vi "(PPMS) Manual Build.vi"(11 "Path to VIPB File":path=path "C:/Users/patrick/Documents/GitHub/PPMS-Monitor-and-Control/build support/PPMS Instrument.vipb") -> ()   [LabVIEW 2019]
uses:
  <userlib>/LevyLab/Build Support/ProgressBar/ProgressBar.lvclass
  <vilib>/AppBuilder/AB_API_Simple/Build Specification Version.ctl
  <vilib>/AppBuilder/AB_API_Simple/Set Build Specification Version (path).vi
  <vilib>/AppBuilder/AB_API_Simple/Build (path).vi
  <vilib>/AppBuilder/AB_API_Simple/NI_App_Builder_API.lvlib
  <vilib>/JKI/VIPM API/VIPM API_vipm_api.lvlib
  <userlib>/LevyLab/Build Support/PostBuildSupport/PostBuildSupport.lvclass
panel:
  out "Current State":string="Exit"
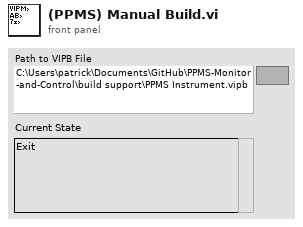
[diagram p1: front panel]
types:
  T1 = enum32{"Invalid", "Standard", "Closed", "Hidden", "Minimized", "Maximized"}
  T2 = enum32{"invalid app kind", "Development System", "Run Time System", "Student Edition", "Embedded LabVIEW", "Evaluation", "Custom"}
  T3 = typedef "NI_App_Builder_API.lvlib/Build Specification Version.ctl" = cluster{"Major":u16, "Minor":u16, "Fix":u16, "Build":u16}
  T4 = cluster{"Core":cluster{"Current VI Reference":refnum<vi>, "Close Panel on Exit?":bool}, "ProgressBar":refnum<class "ProgressBar.lvclass">, "Product Name":string, "Package Version":string, "Package Source Folder":path, "Path to Project":path, "Path to VIPB File":path, "Output Package File Path":path}
  T5 = cluster{"Current VI Reference":refnum<vi>, "Close Panel on Exit?":bool}
  T6 = typedef "VIPM API_vipm_api.lvlib/VI Package Build Spec Data Cluster_vipm_api.ctl" = cluster{"Package Version":T7, "Product Name":string, "Company Name":string, "Author Name (Person or Company)":string, "Product Homepage (URL)":string, "Legal Copyright":string, "License Agreement Name":string, "Product Description Summary":string, "Product Description":string, "Release Notes - Change Log":string}
  T7 = typedef "VIPM API_vipm_api.lvlib/Version Info Cluster_vipm_api.ctl" = cluster{"major":u32, "minor":u32, "patch":u32, "build":u32}
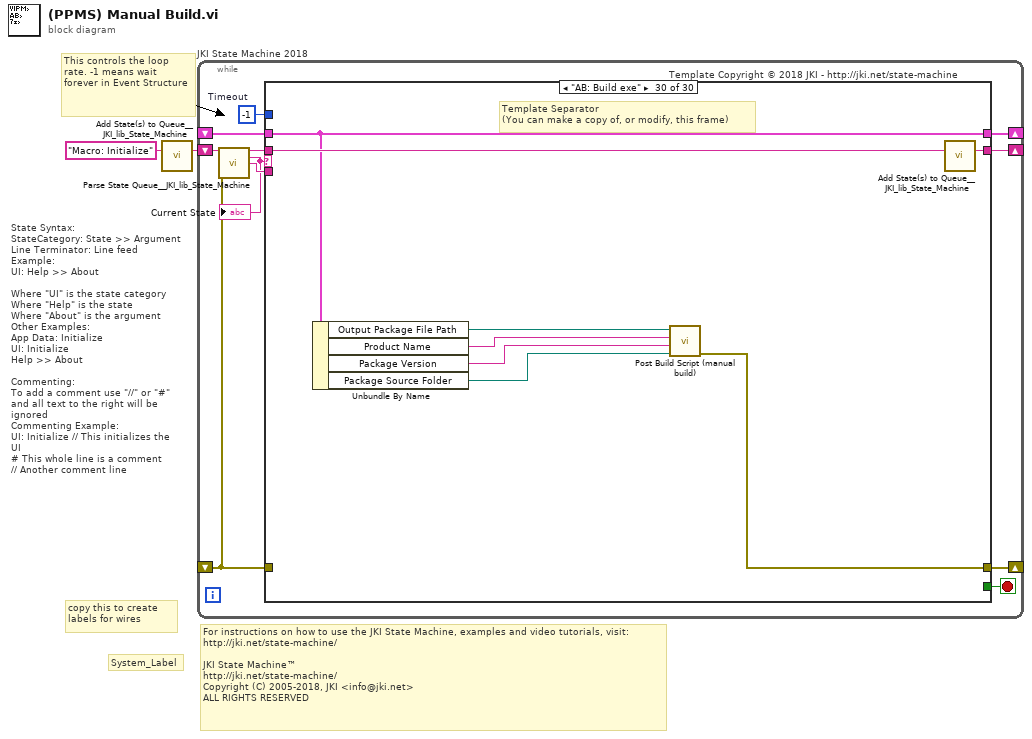
[diagram p0: block diagram]
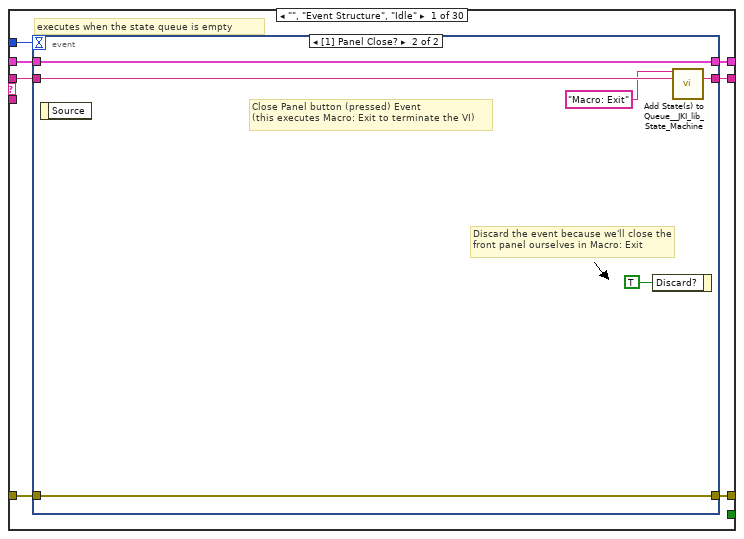
[diagram p2: hidden frame]
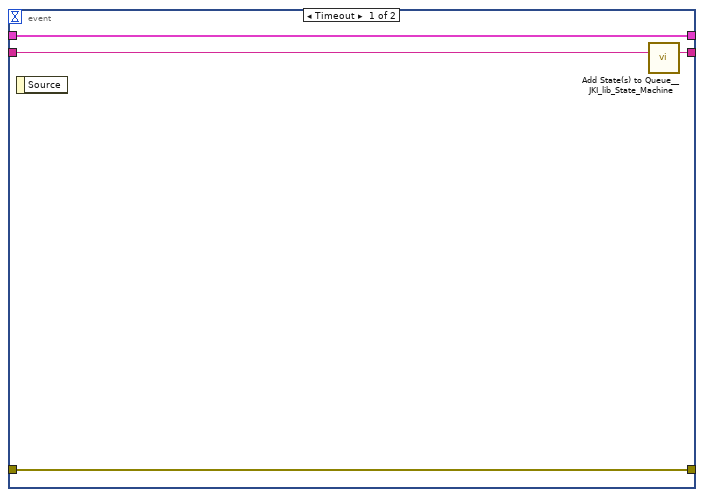
[diagram p3: hidden frame]
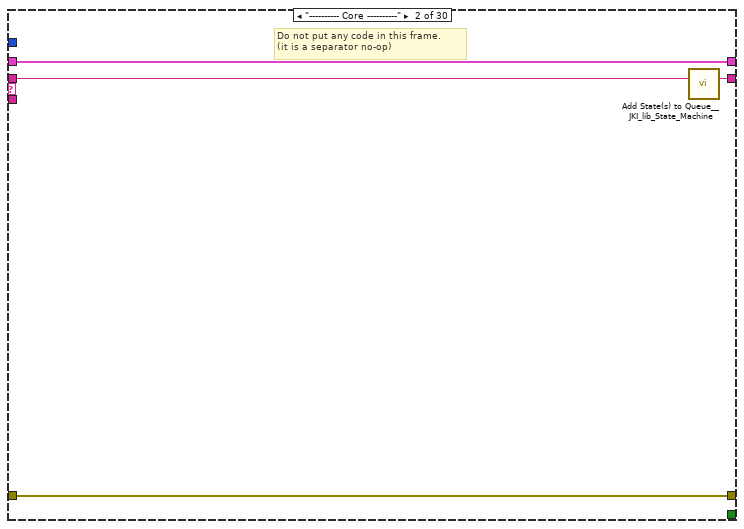
[diagram p4: hidden frame]
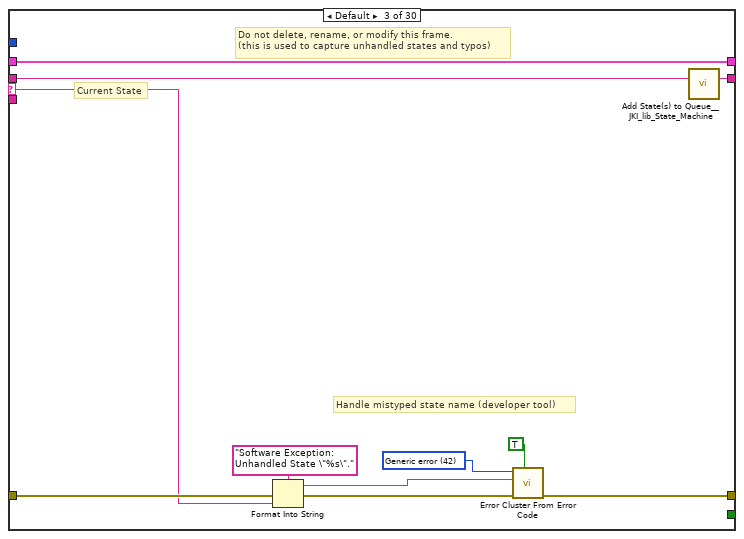
[diagram p5: hidden frame]
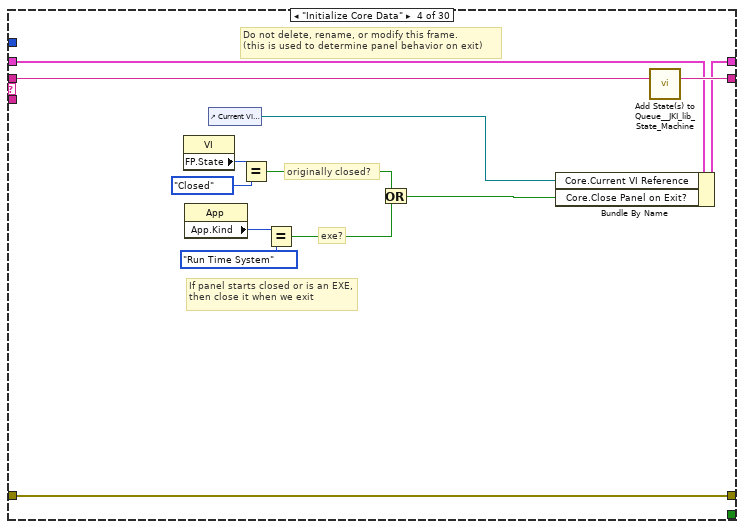
[diagram p6: hidden frame]
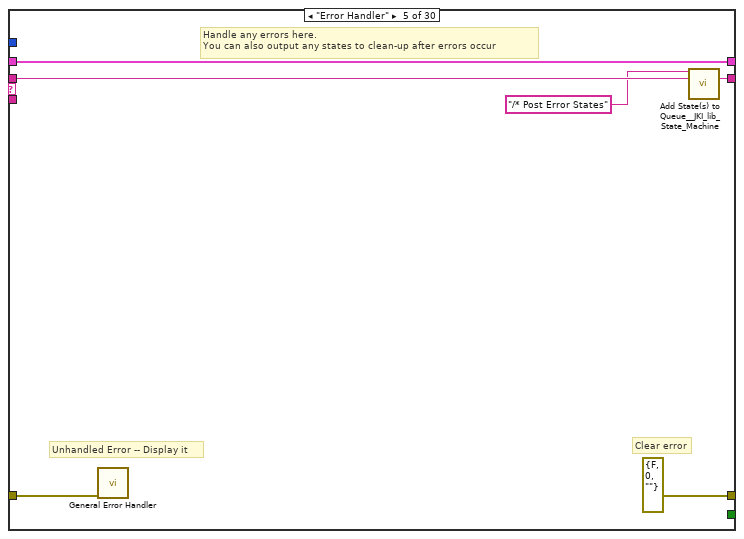
[diagram p7: hidden frame]
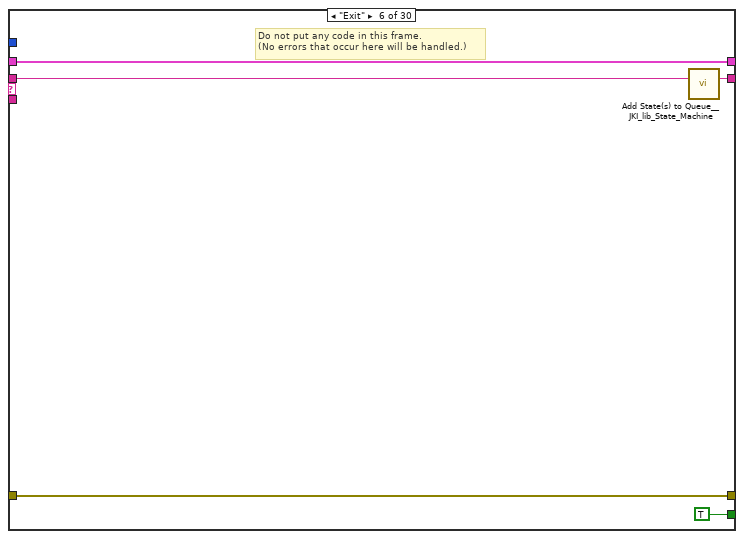
[diagram p8: hidden frame]
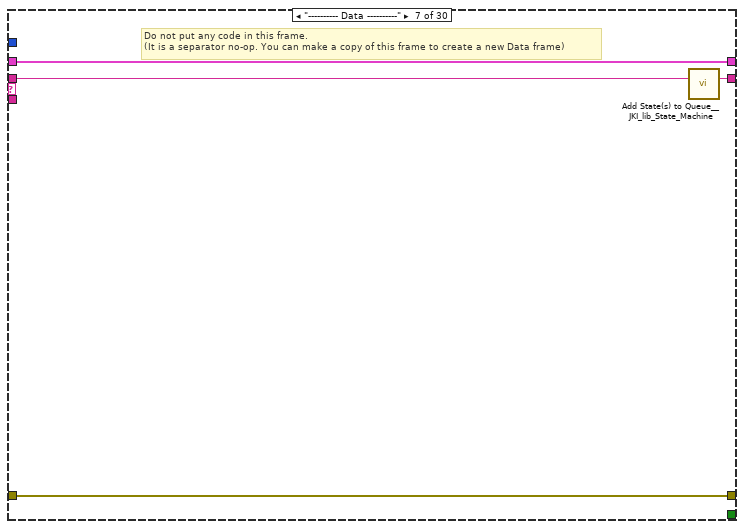
[diagram p9: hidden frame]
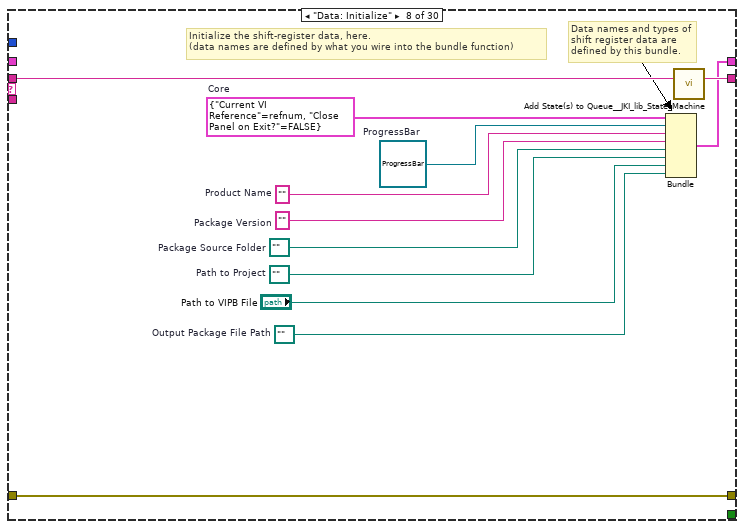
[diagram p10: hidden frame]
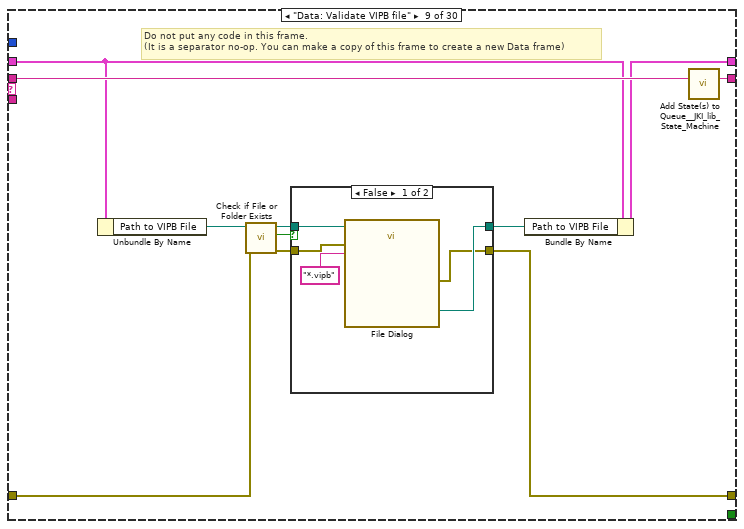
[diagram p11: hidden frame]
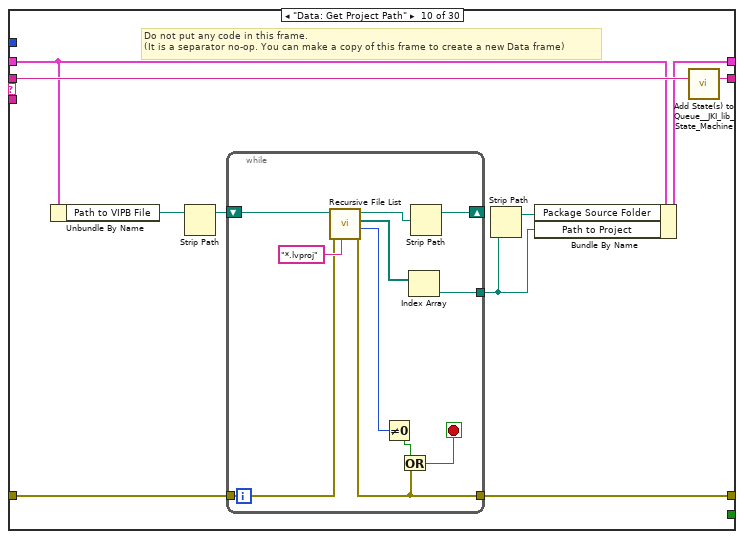
[diagram p13: hidden frame]
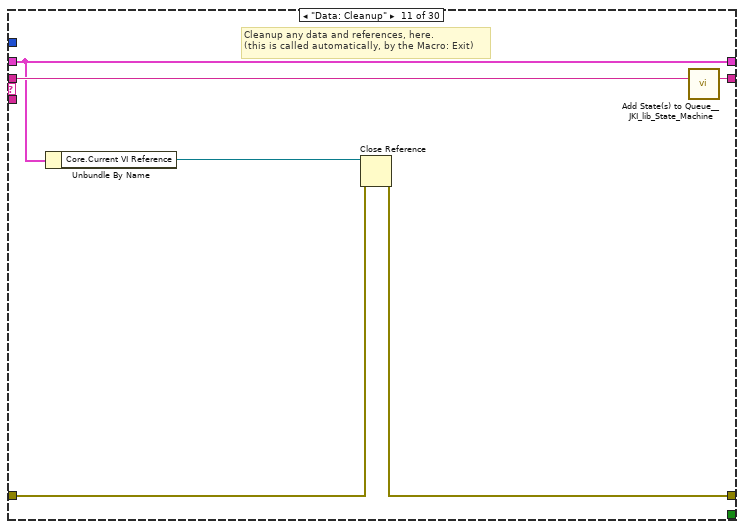
[diagram p14: hidden frame]
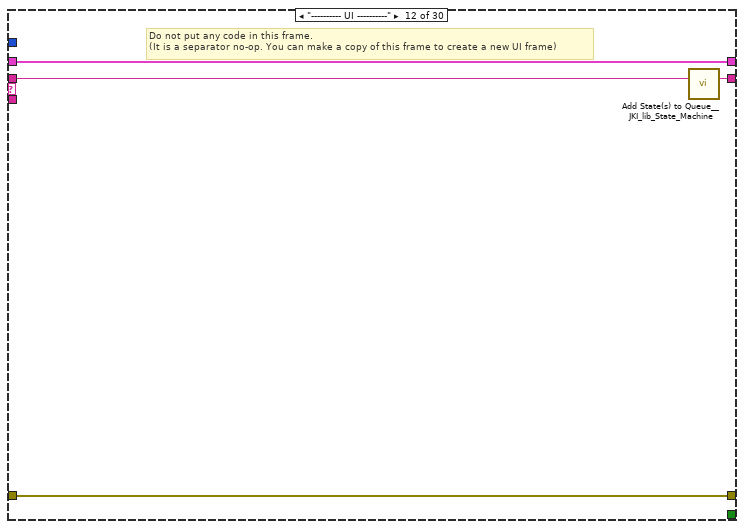
[diagram p15: hidden frame]
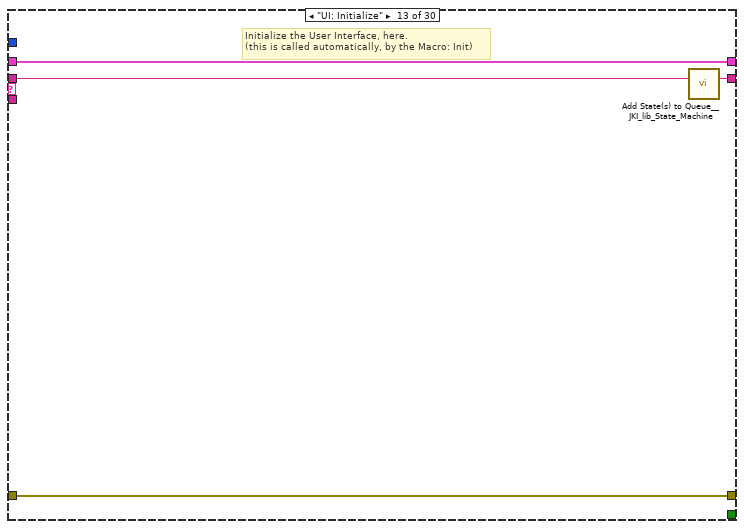
[diagram p16: hidden frame]
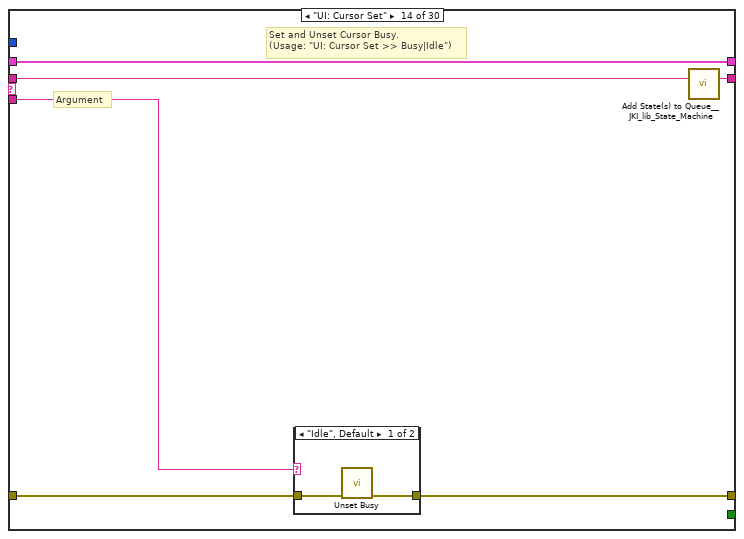
[diagram p17: hidden frame]
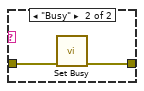
[diagram p18: hidden frame]
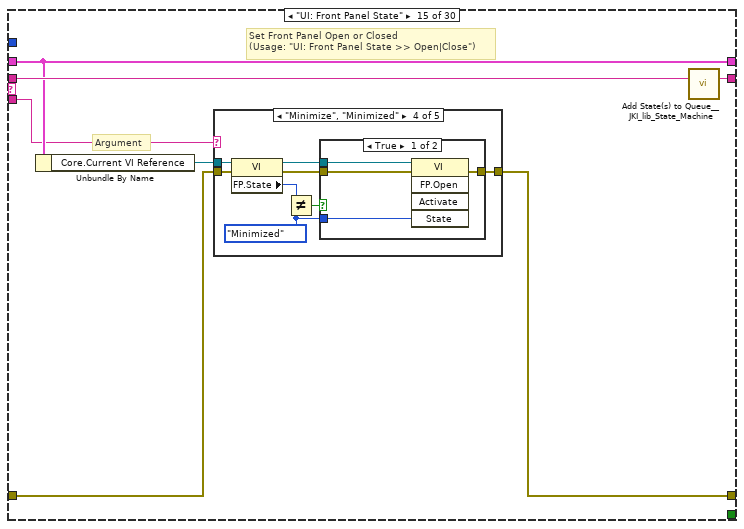
[diagram p19: hidden frame]
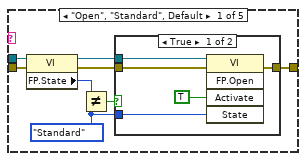
[diagram p20: hidden frame]
diagram:
  # "For instructions on how to use the JKI State Machine, examples and video tutorials, visit:\nhttp://jki.net/state-machine/\n\nJKI State Machine™\nhttp://jki.net/state-machine/\nCopyright (C) 2005-2018, JKI <info@jki.net>\nALL RIGHTS RESERVED"
  # "State Syntax:\nStateCategory: State >> Argument\nLine Terminator: Line feed\nExample:\nUI: Help >> About\n\nWhere \"UI\" is the state category\nWhere \"Help\" is the state\nWhere \"About\" is the argument\nOther Examples:\nApp Data: Initialize\nUI: Initialize\nHelp >> About\n\nCommenting:\nTo add a comment use \"//\" or \"#\" and all text to the right will be ignored\nCommenting Example:\nUI: Initialize // This initializes the UI\n# This whole line is a comment\n// Another comment line"
  # "copy this to create labels for wires"
  # "This controls the loop rate. -1 means wait forever in Event Structure"
  # "System_Label"
  n1 = call <vilib>:"Add State(s) to Queue__JKI_lib_State_Machine.vi"("State(s) in (\"\")"="Macro: Initialize") -> ("States Out"=w2:string)  [unwired: 14 in]
  n2 = while "JKI State Machine 2018" {
    shift-right: [w7] -> _
    shift-left: _ -> [w6]
    shift-right: [w10] -> _
    shift-left: _ -> [w4]
    shift-right: [w9] -> _
    shift-left: w2 -> [w11]
    stop <- w8 stop-if-true
    w5 = -1  # Timeout
    # "Template Copyright © 2018 JKI - http://jki.net/state-machine"
    n3 = call <vilib>:"Parse State Queue__JKI_lib_State_Machine.vi"("State Queue"=w11, "Error In (no error)"=w4) -> ("Remaining States"=w13:string, "Current State"=w3:string, "Arguments"=w12:string)  [unwired: 11 in]
    "Current State" <- w3
    n4 = case shown="\"AB: Build exe\"" w3 {
      selector: w3 -> [_ _ w35 _ _ _ _ _ _ _ _ _ _ _ _ _ _ _ _ _ _ _ _ _ _ _ _ _ w327 _]
      tunnel: w13 -> [w20 w34 w39 w58 w64 w69 w73 w85 w96 w113 w130 w134 w138 w144 w155 w224 w229 w234 w245 w249 w265 w273 w277 w285 w293 w302 w306 w324 w337 w345]
      tunnel: w12 -> [_ _ _ _ _ _ _ _ _ _ _ _ _ w139 w149 _ _ _ _ _ _ _ _ _ _ w294 _ w319 w328 _]
      tunnel: w6 -> [w18 w31 w37 w51 w61 w67 w70 _ w89 w110 w125 w131 w136 w142 w151 w221 w226 w231 w242 w247 w255 w266 w275 w278 w290 w299 w304 w322 w335 w343]
      tunnel: [w17 w32 w41 w55 errorcluster {"status"=FALSE, "code"=0, "source"=""} ("error out") w66 w71 w82 w88 w109 w126 w132 w135 w140 w152 w222 w227 w232 w243 w246 w252 w270 w274 w281 w286 w296 w303 w309 w332 w339] -> w10
      tunnel: w4 -> [w16 w32 w40 w55 w60 w66 w71 w82 w86 w108 w127 w132 w135 w141 w153 w222 w227 w232 w243 w246 w254 w269 w274 w280 w287 w295 w303 w307 w330 _]
      tunnel: [w19 w33 w38 w57 w63 w68 w72 w84 w95 w112 w129 w133 w137 w143 w154 w223 w228 w233 w244 w248 w264 w272 w276 w284 w292 w301 w305 w323 w336 w344] -> w9
      tunnel: [_ _ _ _ _ TRUE _ _ _ _ _ _ _ _ _ _ _ _ _ _ _ _ _ _ _ _ _ _ _ _] -> w8
      tunnel: [w15 w31 w37 w56 w61 w67 w70 w83 w90 w111 w125 w131 w136 w142 w151 w221 w226 w231 w242 w247 w256 w267 w275 w279 w291 w300 w304 w322 w335 w343] -> w7
      tunnel: w5 -> [w14 _ _ _ _ _ _ _ _ _ _ _ _ _ _ _ _ _ _ _ _ _ _ _ _ _ _ _ _ _]
      frame "", "Event Structure", "Idle" {
        # "executes when the state queue is empty"
        n5 = event shown="[1] Panel Close?" {
          selector: _ -> [_ _]
          dyn-events: _ -> [_ _]
          timeout: w14 -> [_ _]
          tunnel: w20 -> [w24 w30]
          tunnel: [w23 w29] -> w19
          tunnel: w18 -> [w21 w27]
          tunnel: [w22 w28] -> w17
          tunnel: w16 -> [w22 w28]
          tunnel: [w21 w27] -> w15
          event Timeout {
            n6 = event-data() -> ()  [unwired: 1 in, 1 out]
            n7 = call <vilib>:"Add State(s) to Queue__JKI_lib_State_Machine.vi"("State(s) in (\"\")"=w24) -> ("States Out"=w23:string)  [unwired: 14 in]
          }
          event Panel Close? {
            # "Discard the event because we'll close the front panel ourselves in Macro: Exit"
            # "Close Panel button (pressed) Event\n(this executes Macro: Exit to terminate the VI)"
            n8 = event-data() -> ()  [unwired: 1 in, 1 out]
            n9 = event-data("Discard?"=TRUE) -> ()  [unwired: 1 in, 1 out]
            n10 = call <vilib>:"Add State(s) to Queue__JKI_lib_State_Machine.vi"("State(s) in Front (\"\")"="Macro: Exit", "State(s) in (\"\")"=w30) -> ("States Out"=w29:string)  [unwired: 13 in]
          }
        }
      }
      frame "---------- Core ----------" {
        # "Do not put any code in this frame.\n(it is a separator no-op)"
        n11 = call <vilib>:"Add State(s) to Queue__JKI_lib_State_Machine.vi"("State(s) in (\"\")"=w34) -> ("States Out"=w33:string)  [unwired: 14 in]
      }
      frame Default {
        w44 = 42 items=["No error", "Argument error", "Memory is full", "Out of zone", "End of file", "File already open", "Generic file I/O error", "File not found", "File permission error", "Disk is full", "Duplicate path", "Too many files open", "System feature not enabled", "Resource file not found", "Cannot add resource", "Resource not found", "Image not found", "Image memory error", "Pen does not exist", "Config type invalid", "Config token not found", "Config parse error", "Config memory error", "Bad external code format", "Bad external code offset", "External code not present", "Null window", "Destroy window error", "Null menu", "Print aborted", "Bad print record", "Print driver error", "Windows error during printing", "Memory error during printing", "Print dialog error", "Generic print error", "Invalid device refnum", "Device not found", "Device parameter error", "Device unit error", "Cannot open device", "Device call aborted", "Generic error", "Cancelled by user", "Object ID too low", "Object ID too high", "Object not in heap", "Unknown heap", "Unknown object (invalid DefProc)", "Unknown object (DefProc not in table)", "Message out of range", "Invalid (null) method", "Unknown message", "Manager call not supported", "Bad address", "Network operation in progress", "Network operation timed out", "Connection is busy", "Network attribute not supported", "Network error", "Address in use", "System out of memory", "Connection aborted", "Connection refused", "Not connected", "Already connected", "Connection closed", "Initialization error (interapplication manager)", "Bad occurrence", "Wait on unbound occurrence handler", "Occurrence queue overflow", "Datalog type conflict", "Unused", "Unrecognized type (interapplication manager)", "Memory corrupt", "Failed to make temporary DLL", "Old CIN version", "Drag socket not found", "Failed to load drop-object", "Failed to register OLE object", "Failed to release OLE object", "Format specifier type mismatch", "Unknown format specifier", "Too few format specifiers", "Too many format specifiers", "Scan failed", "Newer CIN version", "Error converting to variant", "Runtime menu error", "Password tampered", "Variant attribute not found", "Incompatible variant data type", "Event data is not available", "Event Store is not present", "Occurrence is not found", "Event Queue is not created", "Event info is not available", "Refnum passed is NULL", "Error retrieving Class GUID", "Error retrieving CoClass GUID", "Error retrieving TypeLib GUID.", "Bad built application magic bytes.", "Specific driver is different from the specific driver associated with the Logical Name.", "There is no session opened to the class driver.", "Max Error", "MAX - Error with config objects", "MAX - Error loading configuration", "MAX - Group not supported"]
        # "Current State"
        # "Do not delete, rename, or modify this frame.\n(this is used to capture unhandled states and typos)"
        # "Handle mistyped state name (developer tool)"
        n12 = Format Into String(format string="Software Exception: Unhandled State \"%s\"." ("message"), error in=w40, w35) -> (resulting string=w43:string, error out=w42:errorcluster)  [unwired: 1 in]
        n13 = call <vilib>:"Error Cluster From Error Code.vi"("show call chain? (False)"=TRUE, "error in (no error)"=w42, "error message (\"\")"=w43, "error code (0)"=w44) -> ("error out"=w41:errorcluster)  [unwired: 5 in]
        n14 = call <vilib>:"Add State(s) to Queue__JKI_lib_State_Machine.vi"("State(s) in (\"\")"=w39) -> ("States Out"=w38:string)  [unwired: 14 in]
      }
      frame "Initialize Core Data" {
        # "Do not delete, rename, or modify this frame.\n(this is used to determine panel behavior on exit)"
        # "originally closed?"
        # "exe?"
        # "If panel starts closed or is an EXE, then close it when we exit"
        n15 = property class="VI"() -> ("FP.State"=w48:T1)  [unwired: 2 in, 2 out]
        n16 = property class="App"() -> ("App.Kind"=w54:T2)  [unwired: 2 in, 2 out]
        n17 = control-ref of="Current VI Reference"() -> (w49:refnum<vi>)
        n18 = Equal?(x=w48, y=T1."Closed" ("Front Panel Window:State")) -> (x = y?=w46:bool)
        n19 = Equal?(x=w54, y=T2."Run Time System" ("Application:Kind")) -> (x = y?=w52:bool)
        n20 = Or(x=w46, y=w52) -> (x .or. y?=w50:bool)
        n21 = Bundle By Name(cluster=w51, "Core.Current VI Reference"=w49, "Core.Close Panel on Exit?"=w50) -> (w56:T4)
        n22 = call <vilib>:"Add State(s) to Queue__JKI_lib_State_Machine.vi"("State(s) in (\"\")"=w58) -> ("States Out"=w57:string)  [unwired: 14 in]
      }
      frame "Error Handler" {
        # "Unhandled Error -- Display it"
        # "Handle any errors here.\nYou can also output any states to clean-up after errors occur"
        # "Clear error"
        n23 = call <vilib>:"General Error Handler.vi"("error in (no error)"=w60) -> ()  [unwired: 10 in, 5 out]
        n24 = call <vilib>:"Add State(s) to Queue__JKI_lib_State_Machine.vi"("State(s) in Front (\"\")"="/* Post Error States", "State(s) in (\"\")"=w64) -> ("States Out"=w63:string)  [unwired: 13 in]
      }
      frame "Exit" {
        # "Do not put any code in this frame.\n(No errors that occur here will be handled.)"
        n25 = call <vilib>:"Add State(s) to Queue__JKI_lib_State_Machine.vi"("State(s) in (\"\")"=w69) -> ("States Out"=w68:string)  [unwired: 14 in]
      }
      frame "---------- Data ----------" {
        # "Do not put any code in this frame.\n(It is a separator no-op. You can make a copy of this frame to create a new Data frame)"
        n26 = call <vilib>:"Add State(s) to Queue__JKI_lib_State_Machine.vi"("State(s) in (\"\")"=w73) -> ("States Out"=w72:string)  [unwired: 14 in]
      }
      frame "Data: Initialize" {
        w75 = path ""  # Path to Project
        w76 = refnum<class "ProgressBar.lvclass"> refnum  # ProgressBar
        w77 = path ""  # Output Package File Path
        w79 = ""  # Package Version
        w80 = ""  # Product Name
        w78 = path ""  # Package Source Folder
        w81 = T5 {"Current VI Reference"=refnum, "Close Panel on Exit?"=FALSE}  # Core
        # "Data names and types of shift register data are defined by this bundle."
        # "Initialize the shift-register data, here.\n(data names are defined by what you wire into the bundle function)"
        n27 = Bundle("Core"=w81, "ProgressBar"=w76, "Product Name"=w80, "Package Version"=w79, "Package Source Folder"=w78, "Path to Project"=w75, "Path to VIPB File"="Path to VIPB File", "Output Package File Path"=w77) -> (w83:T4)  [unwired: 1 in]
        n28 = call <vilib>:"Add State(s) to Queue__JKI_lib_State_Machine.vi"("State(s) in (\"\")"=w85) -> ("States Out"=w84:string)  [unwired: 14 in]
      }
      frame "Data: Validate VIPB file" {
        # "Do not put any code in this frame.\n(It is a separator no-op. You can make a copy of this frame to create a new Data frame)"
        n29 = Unbundle By Name(w89) -> ("Path to VIPB File"=w93:path)
        n30 = call <vilib>:"Check if File or Folder Exists.vi"("error in (no error)"=w86, "path"=w93) -> ("error out"=w87:errorcluster, "file or folder exists?"=w94:bool, "dup path"=w92:path)  [unwired: 7 in]
        n31 = case shown="False" w94 {
          tunnel: w92 -> [w101 w103]
          tunnel: [w100 w103] -> w91
          tunnel: [w97 w102] -> w88
          tunnel: w87 -> [w99 w102]
          frame False {
            n32 = call "File Dialog"("start path"=w101, "error in"=w99, "pattern (all files)"="*.vipb") -> ("selected path"=w100:path, "error out"=w97:errorcluster)  [unwired: 9 in, 2 out]
          }
          frame True {
          }
        }
        n33 = Bundle By Name(cluster=w89, "Path to VIPB File"=w91) -> (w90:T4)
        n34 = call <vilib>:"Add State(s) to Queue__JKI_lib_State_Machine.vi"("State(s) in (\"\")"=w96) -> ("States Out"=w95:string)  [unwired: 14 in]
      }
      frame "Data: Get Project Path" {
        # "Do not put any code in this frame.\n(It is a separator no-op. You can make a copy of this frame to create a new Data frame)"
        n35 = Unbundle By Name(w110) -> ("Path to VIPB File"=w107:path)
        n36 = Strip Path(path=w107) -> (stripped path=w106:path)  [unwired: 1 out]
        n37 = while {
          tunnel: [w117] -> w109
          tunnel: w108 -> [w119]
          shift-right: [w122] -> _
          shift-left: w106 -> [w118]
          tunnel: [w120] -> w105
          stop <- w115 stop-if-true
          n38 = call <vilib>:"Recursive File List.vi"("pattern"="*.lvproj", "error in (no error)"=w119, "Folder Path"=w118) -> ("error out"=w117:errorcluster, "Number of Files"=w123:i32, "All Files in Dir"=w114:path[], "dup Folder Path"=w121:path)  [unwired: 4 in, 1 out]
          n39 = Not Equal To 0?(x=w123) -> (x != 0?=w116:bool)
          n40 = Or(x=w116, y=w117) -> (x .or. y?=w115:bool)
          n41 = Index Array(array=w114) -> (element=w120:path)  [unwired: 1 in]
          n42 = Strip Path(path=w121) -> (stripped path=w122:path)  [unwired: 1 out]
        }
        n43 = Strip Path(path=w105) -> (stripped path=w104:path)  [unwired: 1 out]
        n44 = Bundle By Name(cluster=w110, "Package Source Folder"=w104, "Path to Project"=w105) -> (w111:T4)
        n45 = call <vilib>:"Add State(s) to Queue__JKI_lib_State_Machine.vi"("State(s) in (\"\")"=w113) -> ("States Out"=w112:string)  [unwired: 14 in]
      }
      frame "Data: Cleanup" {
        # "Cleanup any data and references, here.\n(this is called automatically, by the Macro: Exit)"
        n46 = Unbundle By Name(w125) -> ("Core.Current VI Reference"=w128:refnum<vi>)
        n47 = Close Reference(reference=w128, error in (no error)=w127) -> (error out=w126:errorcluster)
        n48 = call <vilib>:"Add State(s) to Queue__JKI_lib_State_Machine.vi"("State(s) in (\"\")"=w130) -> ("States Out"=w129:string)  [unwired: 14 in]
      }
      frame "---------- UI ----------" {
        # "Do not put any code in this frame.\n(It is a separator no-op. You can make a copy of this frame to create a new UI frame)"
        n49 = call <vilib>:"Add State(s) to Queue__JKI_lib_State_Machine.vi"("State(s) in (\"\")"=w134) -> ("States Out"=w133:string)  [unwired: 14 in]
      }
      frame "UI: Initialize" {
        # "Initialize the User Interface, here.\n(this is called automatically, by the Macro: Init)"
        n50 = call <vilib>:"Add State(s) to Queue__JKI_lib_State_Machine.vi"("State(s) in (\"\")"=w138) -> ("States Out"=w137:string)  [unwired: 14 in]
      }
      frame "UI: Cursor Set" {
        # "Argument"
        # "Set and Unset Cursor Busy.\n(Usage: \"UI: Cursor Set >> Busy|Idle\")"
        n51 = case shown="\"Idle\", Default" w139 {
          tunnel: w141 -> [w146 w148]
          tunnel: [w145 w147] -> w140
          frame "Idle", Default {
            n52 = call <vilib>:"Unset Busy.vi"("error in (no error)"=w146) -> ("error out"=w145:errorcluster)  [unwired: 10 in]
          }
          frame "Busy" {
            n53 = call <vilib>:"Set Busy.vi"("error in (no error)"=w148) -> ("error out"=w147:errorcluster)  [unwired: 9 in, 1 out]
          }
        }
        n54 = call <vilib>:"Add State(s) to Queue__JKI_lib_State_Machine.vi"("State(s) in (\"\")"=w144) -> ("States Out"=w143:string)  [unwired: 14 in]
      }
      frame "UI: Front Panel State" {
        # "Argument"
        # "Set Front Panel Open or Closed\n(Usage: \"UI: Front Panel State >> Open|Close\")"
        n55 = Unbundle By Name(w151) -> ("Core.Current VI Reference"=w150:refnum<vi>)
        n56 = case shown="\"Minimize\", \"Minimized\"" w149 {
          tunnel: w153 -> [w161 w176 w187 w200 w213]
          tunnel: [w163 w177 w189 w202 w215] -> w152
          tunnel: w150 -> [w162 w174 w188 w201 w214]
          frame "Open", "Standard", Default {
            w156 = T1."Standard" ("State")
            n57 = property class="VI"(reference=w162, error in=w161) -> (reference out=w159:refnum<vi>, error out=w160:errorcluster, "FP.State"=w158:T1)
            n58 = Not Equal?(x=w158, y=w156) -> (x != y?=w157:bool)
            n59 = case shown="True" w157 {
              tunnel: [w167 w169] -> w163
              tunnel: w160 -> [w166 w169]
              tunnel: w159 -> [w165 _]
              tunnel: w156 -> [w164 _]
              frame True {
                n60 = invoke class="VI" method="FP.Open"(reference=w165, error in=w166, "Activate"=TRUE, "State"=w164) -> (error out=w167:errorcluster)  [unwired: 1 in, 4 out]
              }
              frame False {
              }
            }
          }
          frame "Close", "Closed" {
            n61 = property class="VI"(reference=w174, error in=w176) -> (reference out=w173:refnum<vi>, error out=w175:errorcluster, "FP.State"=w171:T1)
            n62 = Not Equal?(x=w171, y=T1."Closed" ("Front Panel Window:State")) -> (x != y?=w170:bool)
            n63 = case shown="True" w170 {
              tunnel: [w178 w181] -> w177
              tunnel: w175 -> [w178 w180]
              tunnel: w173 -> [_ w179]
              frame False {
              }
              frame True {
                n64 = invoke class="VI" method="FP.Close"(reference=w179, error in=w180) -> (error out=w181:errorcluster)  [unwired: 1 in, 2 out]
              }
            }
          }
          frame "Hidden", "Hide" {
            w182 = T1."Hidden" ("State")
            n65 = property class="VI"(reference=w188, error in=w187) -> (reference out=w185:refnum<vi>, error out=w186:errorcluster, "FP.State"=w184:T1)
            n66 = Not Equal?(x=w184, y=w182) -> (x != y?=w183:bool)
            n67 = case shown="True" w183 {
              tunnel: [w193 w194] -> w189
              tunnel: w186 -> [w192 w194]
              tunnel: w185 -> [w191 _]
              tunnel: w182 -> [w190 _]
              frame True {
                n68 = invoke class="VI" method="FP.Open"(reference=w191, error in=w192, "State"=w190) -> (error out=w193:errorcluster)  [unwired: 2 in, 4 out]
              }
              frame False {
              }
            }
          }
          frame "Minimize", "Minimized" {
            w195 = T1."Minimized" ("State")
            n69 = property class="VI"(reference=w201, error in=w200) -> (reference out=w198:refnum<vi>, error out=w199:errorcluster, "FP.State"=w197:T1)
            n70 = Not Equal?(x=w197, y=w195) -> (x != y?=w196:bool)
            n71 = case shown="True" w196 {
              tunnel: [w206 w207] -> w202
              tunnel: w199 -> [w205 w207]
              tunnel: w198 -> [w204 _]
              tunnel: w195 -> [w203 _]
              frame True {
                n72 = invoke class="VI" method="FP.Open"(reference=w204, error in=w205, "State"=w203) -> (error out=w206:errorcluster)  [unwired: 2 in, 4 out]
              }
              frame False {
              }
            }
          }
          frame "Maximize", "Maximized" {
            w208 = T1."Maximized" ("State")
            n73 = property class="VI"(reference=w214, error in=w213) -> (reference out=w211:refnum<vi>, error out=w212:errorcluster, "FP.State"=w210:T1)
            n74 = Not Equal?(x=w210, y=w208) -> (x != y?=w209:bool)
            n75 = case shown="True" w209 {
              tunnel: [w219 w220] -> w215
              tunnel: w212 -> [w218 w220]
              tunnel: w211 -> [w217 _]
              tunnel: w208 -> [w216 _]
              frame True {
                n76 = invoke class="VI" method="FP.Open"(reference=w217, error in=w218, "State"=w216) -> (error out=w219:errorcluster)  [unwired: 2 in, 4 out]
              }
              frame False {
              }
            }
          }
        }
        n77 = call <vilib>:"Add State(s) to Queue__JKI_lib_State_Machine.vi"("State(s) in (\"\")"=w155) -> ("States Out"=w154:string)  [unwired: 14 in]
      }
      frame "---------- Macro ----------" {
        # "Do not put any code in this frame.\n(It is a separator no-op. You can make a copy of this frame to create a new Macro frame)"
        n78 = call <vilib>:"Add State(s) to Queue__JKI_lib_State_Machine.vi"("State(s) in (\"\")"=w224) -> ("States Out"=w223:string)  [unwired: 14 in]
      }
      frame "Macro: Initialize" {
        w225 = "Data: Initialize\nInitialize Core Data\nUI: Initialize\nUI: Front Panel State >> Open\nData: Validate VIPB file\n\nMacro: Build\nMacro: Exit"  # Data: Initialize Initialize Core Data UI: Initialize UI: Front Panel State >> Open Data: Validate VIPB file  Macro: Build Macro: Exit
        # "Initialization Macro\n(This is called once, when the VI starts)"
        n79 = call <vilib>:"Add State(s) to Queue__JKI_lib_State_Machine.vi"("State(s) in Front (\"\")"=w225, "State(s) in (\"\")"=w229) -> ("States Out"=w228:string)  [unwired: 13 in]
      }
      frame "Macro: Build" {
        # "Initialization Macro\n(This is called once, when the VI starts)"
        n80 = call <vilib>:"Add State(s) to Queue__JKI_lib_State_Machine.vi"("State(s) in Front (\"\")"="Data: Get Project Path\nVIPM: Read VIPB\nVIPM: Build\nAB: Update Version >> Application\nAB: Update Version >> Installer\nAB: Build >> Application\nAB: Build >> Installer\nAB: Build exe", "State(s) in (\"\")"=w234) -> ("States Out"=w233:string)  [unwired: 13 in]
      }
      frame "Macro: Exit" {
        # "Exit Macro\n(This is called once, when the VI exits)"
        n81 = Unbundle By Name(w242) -> ("Core.Close Panel on Exit?"=w241:bool)
        n82 = Select(t="UI: Front Panel State >> Close", s=w241, f="") -> (s? t:f=w238:string)
        n83 = call <vilib>:"Add State(s) to Queue__JKI_lib_State_Machine.vi"("State(s) in Front (\"\")"="", "State(s) in (\"\")"=w238, "State(s) at Back (\"\")"="Data: Cleanup\nExit") -> ("States Out"=w236:string)  [unwired: 12 in]
        n84 = call <vilib>:"Add State(s) to Queue__JKI_lib_State_Machine.vi"("State(s) in Front (\"\")"=w236, "State(s) in (\"\")"=w245) -> ("States Out"=w244:string)  [unwired: 13 in]
      }
      frame "---------- VIPM ----------" {
        # "Template Separator\n(You can make a copy of, or modify, this frame)"
        n85 = call <vilib>:"Add State(s) to Queue__JKI_lib_State_Machine.vi"("State(s) in (\"\")"=w249) -> ("States Out"=w248:string)  [unwired: 14 in]
      }
      frame "VIPM: Read VIPB" {
        # "Your code here.\n(You can make a copy of, or modify, this frame)"
        n86 = Unbundle By Name(w255) -> ("Path to VIPB File"=w258:path)
        n87 = call <vilib>:"Read VI Package Build Spec_vipm_api.vi"("error in (no error)"=w254, "Path to VIPB File"=w258) -> ("error out"=w253:errorcluster, "VI Package Build Spec Data"=w263:T6)  [unwired: 8 in]
        n88 = Unbundle By Name(w263) -> ("Package Version.major"=w251:u32, "Package Version.minor"=w262:u32, "Package Version.patch"=w261:u32, "Package Version.build"=w260:u32, "Product Name"=w250:string)
        n89 = Format Into String(format string="%d.%d.%d.%d", error in=w253, w251, w262, w261, w260) -> (resulting string=w257:string, error out=w252:errorcluster)  [unwired: 1 in]
        n90 = Bundle By Name(cluster=w255, "Package Version"=w257, "Product Name"=w250) -> (w256:T4)
        n91 = call <vilib>:"Add State(s) to Queue__JKI_lib_State_Machine.vi"("State(s) in (\"\")"=w265) -> ("States Out"=w264:string)  [unwired: 14 in]
      }
      frame "VIPM: Build" {
        # "Your code here.\n(You can make a copy of, or modify, this frame)"
        n92 = Unbundle By Name(w266) -> ("Path to VIPB File"=w271:path)
        n93 = call <vilib>:"Build VI Package_vipm_api.vi"("error in (no error)"=w269, "Path to VIPB File"=w271) -> ("error out"=w270:errorcluster, "Build Output"=w268:path)  [unwired: 8 in]
        n94 = Bundle By Name(cluster=w266, "Output Package File Path"=w268) -> (w267:T4)
        n95 = call <vilib>:"Add State(s) to Queue__JKI_lib_State_Machine.vi"("State(s) in (\"\")"=w273) -> ("States Out"=w272:string)  [unwired: 14 in]
      }
      frame "---------- ProgressBar ----------" {
        # "Template Separator\n(You can make a copy of, or modify, this frame)"
        n96 = call <vilib>:"Add State(s) to Queue__JKI_lib_State_Machine.vi"("State(s) in (\"\")"=w277) -> ("States Out"=w276:string)  [unwired: 14 in]
      }
      frame "ProgressBar: Initialize" {
        # "Do not put any code in this frame.\n(It is a separator no-op. You can make a copy of this frame to create a new Data frame)"
        n97 = Unbundle By Name(w278) -> ("ProgressBar"=w283:refnum<class "ProgressBar.lvclass">)
        n98 = call <userlib>:"Initialize ProgressBar.vi"("error in (no error)"=w280, "ProgressBar in"=w283) -> ("error out"=w281:errorcluster, "ProgressBar out"=w282:refnum<class "ProgressBar.lvclass">)  [unwired: 8 in]
        n99 = Bundle By Name(cluster=w278, "ProgressBar"=w282) -> (w279:T4)
        n100 = call <vilib>:"Add State(s) to Queue__JKI_lib_State_Machine.vi"("State(s) in (\"\")"=w285) -> ("States Out"=w284:string)  [unwired: 14 in]
      }
      frame "ProgressBar: Destroy" {
        # "Do not put any code in this frame.\n(It is a separator no-op. You can make a copy of this frame to create a new Data frame)"
        n101 = Unbundle By Name(w290) -> ("ProgressBar"=w289:refnum<class "ProgressBar.lvclass">)
        n102 = call <userlib>:"Destroy ProgressBar.vi"("error in (no error)"=w287, "ProgressBar in"=w289) -> ("error out"=w286:errorcluster, "ProgressBar out"=w288:refnum<class "ProgressBar.lvclass">)  [unwired: 8 in]
        n103 = Bundle By Name(cluster=w290, "ProgressBar"=w288) -> (w291:T4)
        n104 = call <vilib>:"Add State(s) to Queue__JKI_lib_State_Machine.vi"("State(s) in (\"\")"=w293) -> ("States Out"=w292:string)  [unwired: 14 in]
      }
      frame "ProgressBar: Update" {
        # "Template Separator\n(You can make a copy of, or modify, this frame)"
        n105 = Unbundle By Name(w299) -> ("ProgressBar"=w298:refnum<class "ProgressBar.lvclass">)
        n106 = call <userlib>:"Send Progress and Message.vi"("error in (no error)"=w295, "Message"=w294, "ProgressBar in"=w298) -> ("error out"=w296:errorcluster, "ProgressBar out"=w297:refnum<class "ProgressBar.lvclass">)  [unwired: 7 in]
        n107 = Bundle By Name(cluster=w299, "ProgressBar"=w297) -> (w300:T4)
        n108 = call <vilib>:"Add State(s) to Queue__JKI_lib_State_Machine.vi"("State(s) in (\"\")"=w302) -> ("States Out"=w301:string)  [unwired: 14 in]
      }
      frame "---------- AB ----------" {
        # "Template Separator\n(You can make a copy of, or modify, this frame)"
        n109 = call <vilib>:"Add State(s) to Queue__JKI_lib_State_Machine.vi"("State(s) in (\"\")"=w306) -> ("States Out"=w305:string)  [unwired: 14 in]
      }
      frame "AB: Update Version" {
        # "Template Separator\n(You can make a copy of, or modify, this frame)"
        n110 = Unbundle By Name(w322) -> ("Path to Project"=w308:path, "Product Name"=w320:string, "Package Version"=w317:string)
        n111 = Format Into String(format string="%s %s", w320, w319) -> (resulting string=w318:string)  [unwired: 2 in, 1 out]
        n112 = Scan From String(format string="%d.%d.%d.%d", input string=w317) -> (output 1=w315:i32, output 2=w312:i32, output 3=w311:i32, output 4=w310:i32)  [unwired: 6 in, 3 out]
        n113 = Bundle By Name(cluster=T3 {"Major"=0, "Minor"=0, "Fix"=0, "Build"=0} ("Build Specification Version"), "Major"=w315, "Minor"=w312, "Fix"=w311, "Build"=w310) -> (w313:T3)
        n114 = call-poly <vilib>:"Set Build Specification Version.vi"("Build Specification Version"=w313, "error in (no error)"=w307, "Name of build specification"=w318, "Path to project"=w308) -> ("error out"=w309:errorcluster)  [unwired: 7 in]
        n115 = call <vilib>:"Add State(s) to Queue__JKI_lib_State_Machine.vi"("State(s) in (\"\")"=w324) -> ("States Out"=w323:string)  [unwired: 14 in]
      }
      frame "AB: Build" {
        # "Template Separator\n(You can make a copy of, or modify, this frame)"
        n116 = Unbundle By Name(w335) -> ("Path to Project"=w331:path, "Product Name"=w333:string)
        n117 = Format Into String(format string="%s %s", w327, w328) -> (resulting string=w326:string)  [unwired: 2 in, 1 out]
        n118 = Format Into String(format string="%s %s", w333, w328) -> (resulting string=w329:string)  [unwired: 2 in, 1 out]
        n119 = local write "Current State"(w326) -> ()
        n120 = call-poly <vilib>:"Build.vi"("error in (no error)"=w330, "Name of build specification (if empty: build all)"=w329, "Path to project"=w331) -> ("error out"=w332:errorcluster)  [unwired: 7 in, 1 out]
        n121 = call <vilib>:"Add State(s) to Queue__JKI_lib_State_Machine.vi"("State(s) in (\"\")"=w337) -> ("States Out"=w336:string)  [unwired: 14 in]
      }
      frame "AB: Build exe" {
        # "Template Separator\n(You can make a copy of, or modify, this frame)"
        n122 = Unbundle By Name(w343) -> ("Output Package File Path"=w342:path, "Product Name"=w340:string, "Package Version"=w338:string, "Package Source Folder"=w341:path)
        n123 = call <userlib>:"Post Build Script (manual build).vi"("Package Source Folder"=w341, "Package Version"=w338, "Product Name"=w340, "Output Package File Path"=w342) -> ("error out"=w339:errorcluster)  [unwired: 7 in]
        n124 = call <vilib>:"Add State(s) to Queue__JKI_lib_State_Machine.vi"("State(s) in (\"\")"=w345) -> ("States Out"=w344:string)  [unwired: 14 in]
      }
    }
  }
